vi "Add Key Dialog.vi"(8 "error in":errorcluster, 11 "Config in":refnum<class "Config.lvclass">) -> (0 "error out":errorcluster, 3 "Config out":refnum<class "Config.lvclass">)   [LabVIEW 2023, in "Config.lvlib" / "Config.lvclass"]
uses:
  Config.lvclass
panel:
  out "Dialog":string
  in  "Cancel Button":bool
  in  "OK Button":bool
  in  "Key Value":string
  in  "Key Name":string
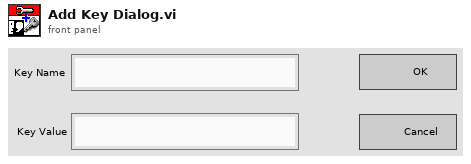
[diagram p1: front panel]
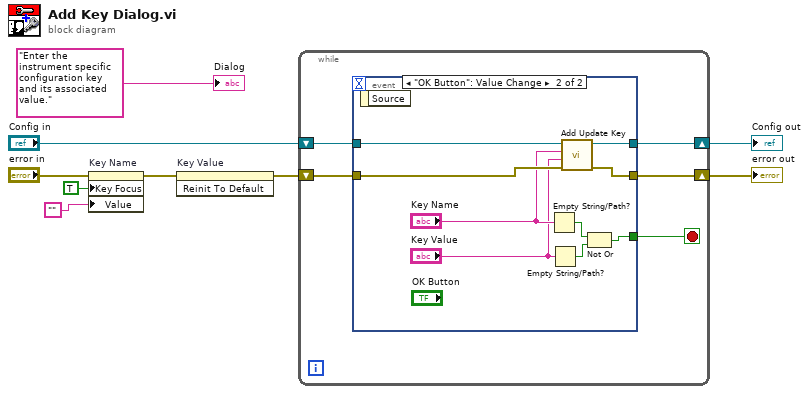
[diagram p0: block diagram]
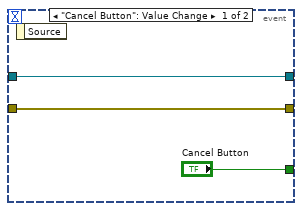
[diagram p2: hidden frame]
diagram:
  n1 = property on="Key Name" class="Str"(error in="error in", "Key Focus"=TRUE, "Value"="") -> (error out=w5:errorcluster)  [unwired: 1 in, 1 out]
  n2 = invoke on="Key Value" class="Str" method="Reinit To Default"(error in=w5) -> (error out=w3:errorcluster)  [unwired: 2 in, 2 out]
  n3 = while {
    shift-right: [w13] -> w8
    shift-left: "Config in" -> [w14]
    shift-right: [w12] -> w7
    shift-left: w3 -> [w11]
    stop <- w10 stop-if-true
    n4 = event shown="[1] \"OK Button\": Value Change" {
      selector: _ -> [_ _]
      dyn-events: _ -> [_ _]
      timeout: _ -> [_ _]
      tunnel: w14 -> [w17 w25]
      tunnel: [w17 w26] -> w13
      tunnel: [w16 w24] -> w12
      tunnel: w11 -> [w16 w23]
      tunnel: ["Cancel Button" w18] -> w10
      event "Cancel Button": Value Change {
        n5 = event-data() -> ()  [unwired: 1 in, 1 out]
      }
      event "OK Button": Value Change {
        n6 = event-data() -> ()  [unwired: 1 in, 1 out]
        n7 = Empty String/Path?(string/path="Key Name") -> (empty?=w19:bool)
        n8 = Empty String/Path?(string/path="Key Value") -> (empty?=w20:bool)
        n9 = call "Add Update Key.vi"("error in"=w23, "Value"="Key Value", "Key"="Key Name", "Config in"=w25) -> ("error out"=w24:errorcluster, "Config out"=w26:refnum<class "Config.lvclass">)  [unwired: 6 in]
        n10 = Not Or(1:w20, 2:w19) -> (0:w18:bool)
      }
    }
  }
  "error out" <- w7
  "Config out" <- w8
  "Dialog" <- "Enter the instrument specific configuration key and its associated value."
